vi "Simulation - Kopie.vi"() -> ()   [LabVIEW 2014]
uses:
  <vilib>/Simulation/Scripting/Companion Diagram/SimConfigNode/SimParams.ctl
  <vilib>/Simulation/Scripting/Companion Diagram/SimConfigNode/_simSolvers.ctl
  <vilib>/Simulation/Implementation/Shared/SIMSCR Execution Mode.ctl
  <vilib>/Platform/TimedLoop/XDataNode/timing_clust.ctl
  <vilib>/Platform/TimedLoop/XDataNode/nitl_modes.ctl
  <vilib>/Platform/TimedLoop/XDataNode/wakeup.ctl
  <vilib>/Simulation/Param Hierarchy/Typedefs/SIMPH Param Control Actions.ctl
  <vilib>/Analysis/3filter.llb/Filter Passband Type.ctl
  <vilib>/Simulation/Implementation/Shared/NILVSim_ParamChanged.vi
  <vilib>/Simulation/Implementation/Shared/NILVSim_FinishedLate.vi
  <vilib>/Simulation/Implementation/Shared/NILVSIM_BeginStep.vi
  <vilib>/Simulation/Utility/Implementation/SIM Halt.vi
  <vilib>/Simulation/SignalArithmetic/Implementation/NILVSim Gain.llb/SIM Gain (scalar).vi
  <vilib>/Simulation/ContinuousLinear/Implementation/NILVSim Transfer Function.llb/SIM Transfer Function Distributor (SISO).vi
  <vilib>/Simulation/Implementation/Shared/SIM Is Init or Final Stage.vi
  <vilib>/Simulation/ContinuousLinear/Implementation/NILVSim State Space.llb/SIM State Space Distributor (CD).vi
  <vilib>/Simulation/Nonlinear/Implementation/NILVSim Quantizer.llb/SIM Quantizer (scalar).vi
  <vilib>/Simulation/ContinuousLinear/Implementation/NILVSim Transfer Function.llb/SIM Transfer Function Collector (SISO).vi
  <vilib>/Simulation/SignalArithmetic/Implementation/NILVSim Gain.llb/SIM Gain (vector,MatrixGain).vi
  <vilib>/Simulation/Nonlinear/Implementation/NILVSim Saturation.llb/SIM Saturation (scalar).vi
  <vilib>/Simulation/ContinuousLinear/Implementation/NILVSim State Space.llb/SIM State Space Collector (CD).vi
  <vilib>/Simulation/SignalArithmetic/Implementation/NILVSim Gain.llb/SIM Gain (vector).vi
  <vilib>/Simulation/Implementation/Shared/NILVSim_Manager.vi
  <vilib>/Utility/error.llb/Clear Errors.vi
  <vilib>/Simulation/Implementation/Shared/NILVSim_FinalizeModel.vi
  <vilib>/addons/Control Design/_Model Construction/Model Creation.llb/Model Creation SubVI/cd_Create State Space Model.vi
  <vilib>/addons/Control Design/_Utility/Model Viewer.llb/Model Viewer SubVI/cd_Draw State-Space Equation (SS).vi
  <vilib>/Simulation/Implementation/Shared/SIM Unbundle Sim Info.vi
  <vilib>/Simulation/Implementation/Shared/SIMSH Read Queue.vi
  <vilib>/Simulation/Implementation/Shared/NILVSim_Initialize.vi
  <vilib>/addons/Control Design/_State Feedback Control/State Feedback Control.llb/CD Linear Quadratic Regulator.vi
  <vilib>/addons/Control Design/_State Feedback Control/State Feedback Control.llb/State Feedback Control SubVis/cd_Linear Quadratic Regulator.vi
  <vilib>/ptbypt/Probability & Statistics.llb/Median PtByPt.vi
  <vilib>/Simulation/Utility/Implementation/NILVSim Get Time and IsAcceptedStep.vi
  <vilib>/ptbypt/Filters.llb/Butterworth Filter PtByPt.vi
  <vilib>/Simulation/Implementation/Shared/NILVSim_GetModelError.vi
  <vilib>/Simulation/Implementation/Shared/SIM Bundle Sim Info.vi
  <vilib>/Simulation/Scripting/Companion Diagram/SimConfigNode/SimDog.xnode
  Nichtlineares Pendelmodell Sub.vi
  LabView/Beobachter/Nichtlinearer Beobachter.vi
  <vilib>/Platform/TimedLoop/XDataNode/XDataNode.xnode
  <vilib>/addons/Control Design/_Model Construction/Model Typedefs.llb/CD State Space Model (MIMO).ctl
  <vilib>/addons/Control Design/_Model Construction/Model Typedefs.llb/CD General Elements.ctl
  <vilib>/Simulation/Implementation/XNodeFramework/SimXNode/SimX.xnode
  <vilib>/addons/Control Design/_Model Construction/NI_LinSys_Model Typedefs.lvlib
  <vilib>/addons/Control Design/_State Feedback Control/NI_CD_State Feedback Control.lvlib
  <vilib>/addons/Control Design/_Utility/NI_CD_Model Viewer.lvlib
  <vilib>/addons/Control Design/_Model Construction/NI_LinSys_Model Creation.lvlib
  <vilib>/Simulation/ContinuousLinear/Implementation/NILVSim State Space.llb/SIM State Space (CD).vi
  <vilib>/ptbypt/NI_PtbyPt.lvlib
  <vilib>/Analysis/NI_AALBase.lvlib
  <vilib>/Simulation/ContinuousLinear/Implementation/NILVSim Transfer Function.llb/SIM Transfer Function (SISO).vi
  <vilib>/Platform/TimedLoop/XDataNode/XDNodeRunTimeDep.lvlib
  <vilib>/Simulation/Implementation/Shared/NI_SIM_Implementation.lvlib
panel:
  in  "Kraftverstärkung":dbl=1.0
  in  "Winkelg._t0":dbl
  in  "Enum":enum16{"median", "kein", "pt2"}(ring)
  in  "Enc. resolution":dbl
  in  "low cutoff freq: fl":dbl=0.125 caption="Untere Grenzfreq: fl" format="%0.3f"
  in  "WG Regler":T1(ring)
  out "Winkelgeschw. geschätzt vs gesch.+gefiltert (abs. Fehler)":dbl(graph)
  in  "WG Aufschw.":T1(ring)
  out "geschätzt+gefiltert":dbl
  out "Cruise mode":i32(graph)=1
  out "Regler":i16(graph)=1
  in  "< Winkelgeschwindigkeit (rad)":dbl=1.0
  in  ">Winkel (Grad) AUS":dbl=15.0
  in  "<Winkel (Grad) EIN":dbl=10.0
  in  "k_eu (EIN)":dbl=0.02
  in  "k_el (AUS)":dbl=-0.1
  in  "k_eo (Energieoffset)":dbl=0.02
  in  "k_ce (Energiezufuhr)":dbl=5.0
  out "E kin":sgl(graph)=9.683897e-12
  out "E pot":sgl(graph)=-2.0909203e-09
  out "E gesamt":sgl(graph)=-2.0812365e-09
  in  "Position_t0 (m)":dbl
  out "Kraft in N":dbl=0.019527387596300915
  out "winkelgesch Geschätzt":dbl=-3.1760654462499827e-05
  out "Winkelgesch. Simuliert":dbl=-3.1760671506439986e-05
  out "Winkel  (rad)":dbl=6.283279545734089
  out "Geschwindigkeit":dbl=-0.0005385174095775639
  out "Position":dbl=-499.86322344217655
  out "Regler EIN":bool=TRUE
  in  "k_v (velocity well)":dbl=1.0
  in  "k_x (cart well)":dbl=2.5
  in  "k_e (Energiezufuhr)":dbl=2.2
  in  "Aufschwingen":bool=TRUE
  in  "Strecke":T2(ring)
  out "State-Space Equation":picture
  out "Position (mm)":cluster{"output":dbl, "output":dbl}(graph)={"output"=-500.0, "output"=-499.86322344217655}
  out "Winkel (Grad)":T3(graph)
  out "Kraft (N)":dbl(graph)=0.019527387596300915
  out "Geschwindigkeit":dbl(graph)=-0.0005385174095775639
  out "Winkelgeschwindigkeit":T4(graph)
  out "K":dbl[][](array[numeric])=[[-100.00000000000013, -103.52787904437508, -700.9266185415707, -140.20536929914581]] format="%.2f"
  in  "Q":dbl[][](array[numeric])=[[100.0, 0.0, 0.0, 0.0], [0.0, 1.0, 0.0, 0.0], [0.0, 0.0, 100.0, 0.0], [0.0, 0.0, 0.0, 1.0]] format="%.2f"
  in  "R":dbl[][](array[numeric])=[[0.01]] format="%.2f"
  in  "Regler":bool=TRUE
  in  "Winkel_t0 (Grad)":dbl=180.0
  in  "Sollwert Amplitude (mm)":dbl=-500.0
  in  "Stop Button":bool
  # "Anfangswerte"
  # "Aufschwingparameter"
  # "Umschalten auf Cruise Mode. Energiegrenzen in J."
  # "Umschalten auf Regler"
  # "LQR Regler"
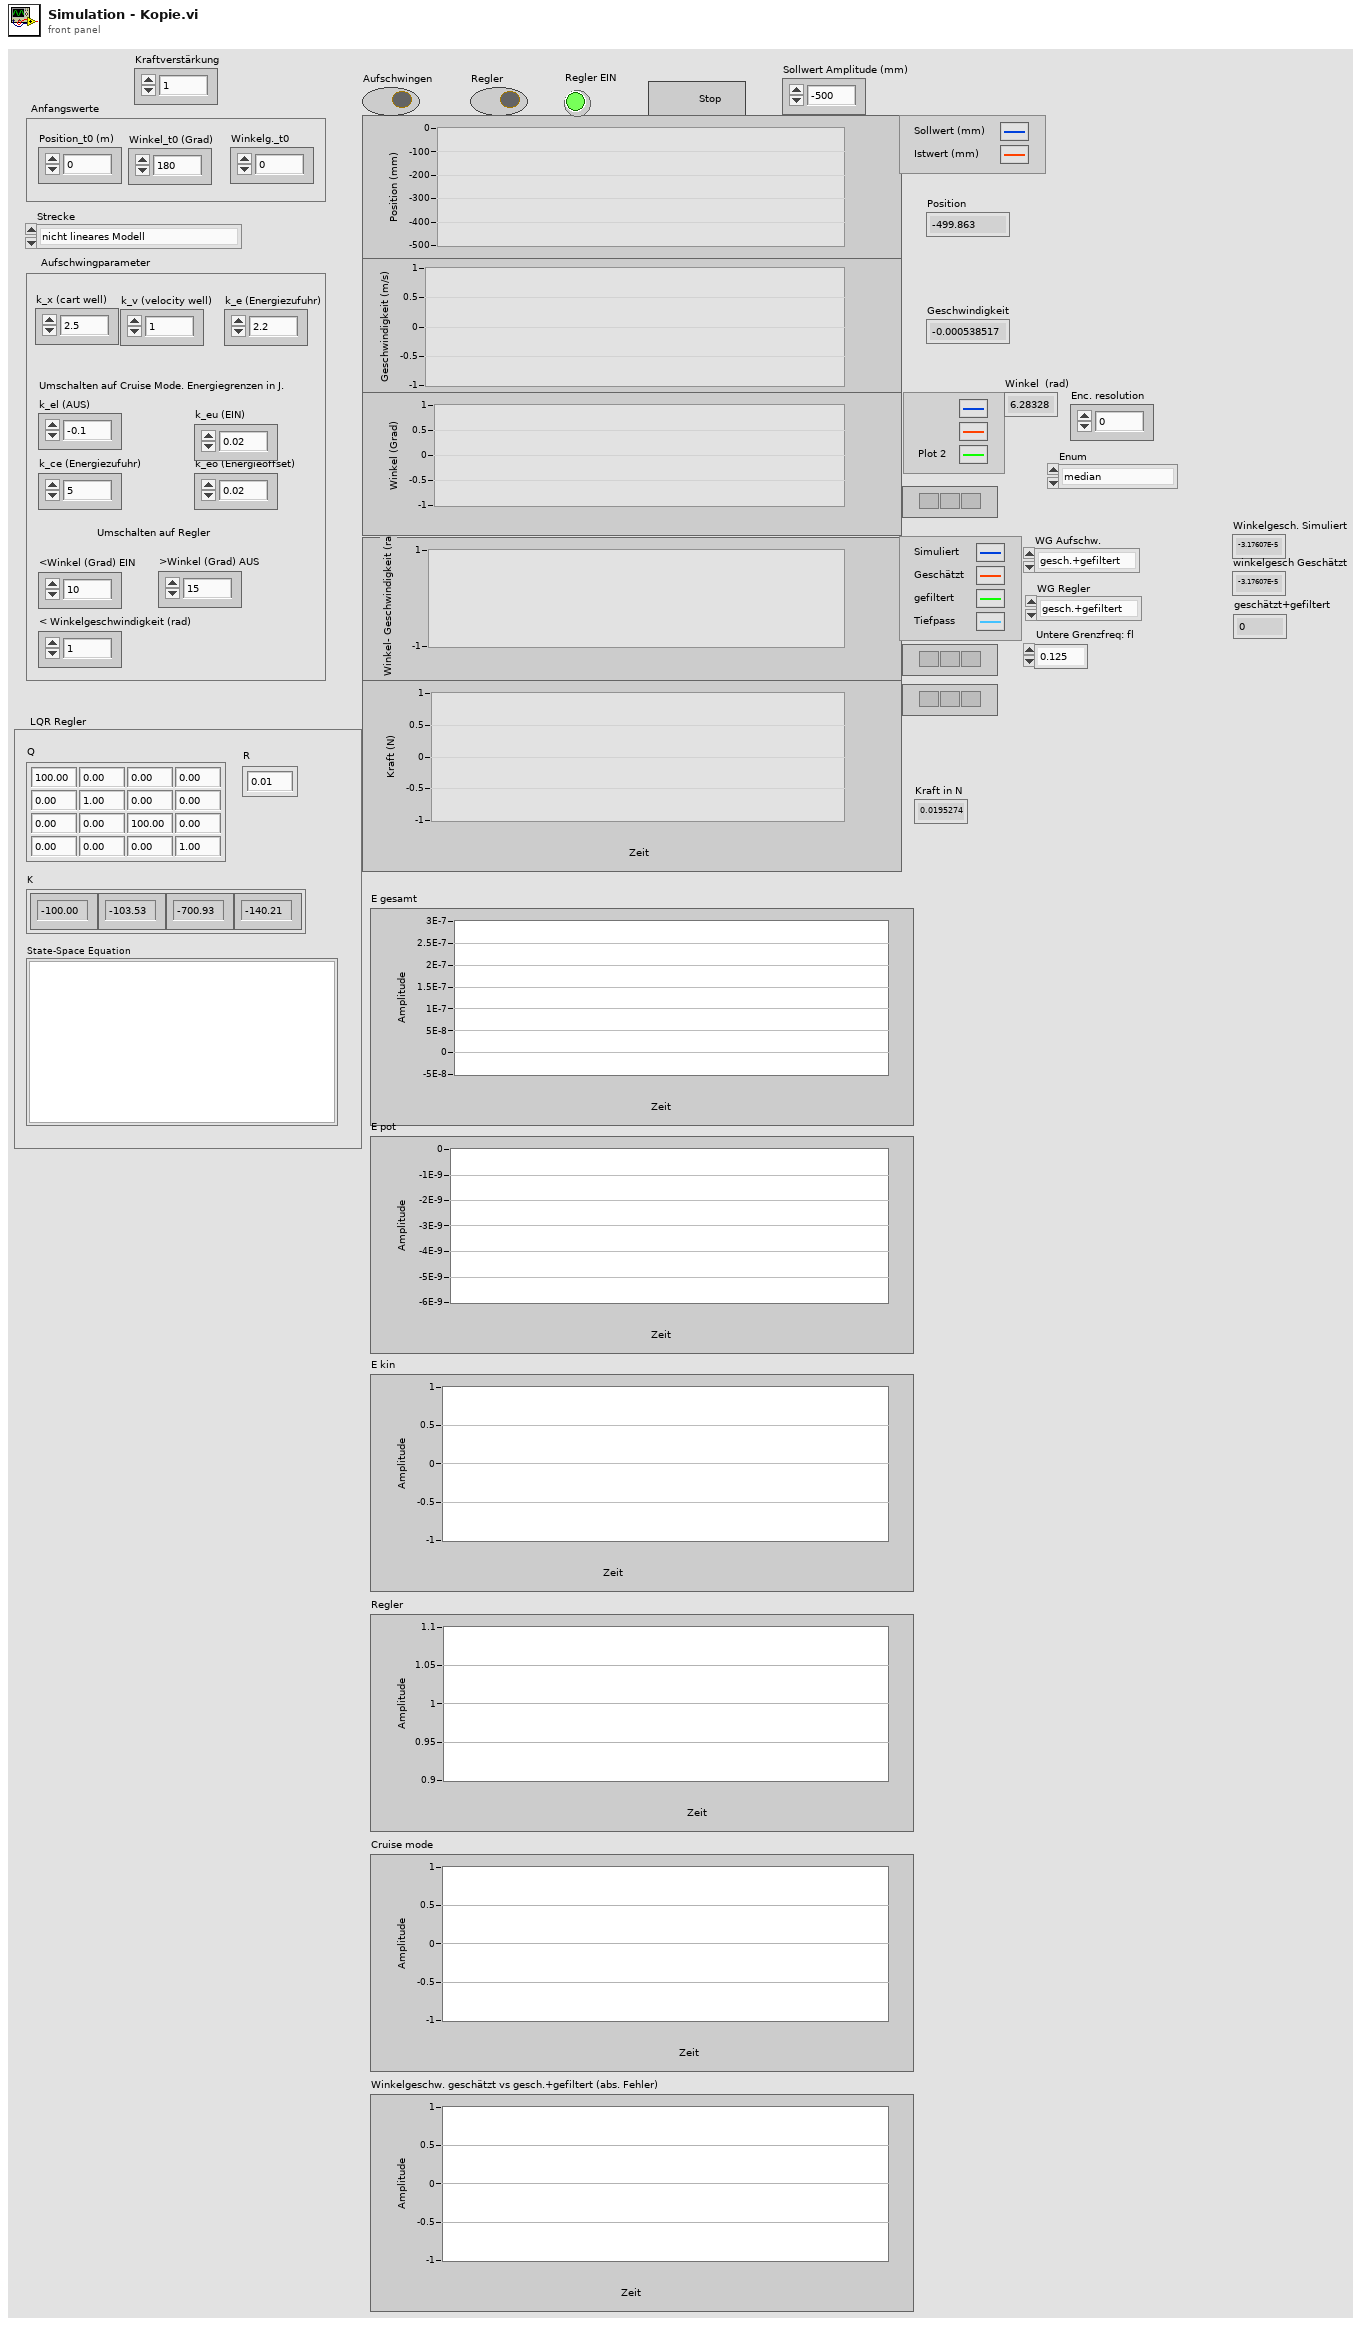
[diagram p1: front panel]
types:
  T1 = enum16{"gesch.+gefiltert", "geschätzt", "simuliert"}
  T2 = enum16{"nicht lineares Modell", "lineares Modell"}
  T3 = cluster{"output":dbl, "output y(t)":dbl, "median":dbl}
  T4 = cluster{"Winkelgesch":dbl, "x4_":dbl, "median":dbl, "Filtered x":dbl}
  T5 = typedef "NI_LinSys_Model Typedefs.lvlib/CD State Space Model (MIMO).ctl" = cluster{"properties":T6, "A":dbl[][], "B":dbl[][], "C":dbl[][], "D":dbl[][], "StateNames":string[], "Transport Delay":dbl[][]}
  T6 = typedef "NI_LinSys_Model Typedefs.lvlib/CD General Elements.ctl" = cluster{"Model name":string, "Input names":string[], "Output names":string[], "Input Delays":dbl[], "Output Delays":dbl[], "Sampling Time":dbl, "Notes":string}
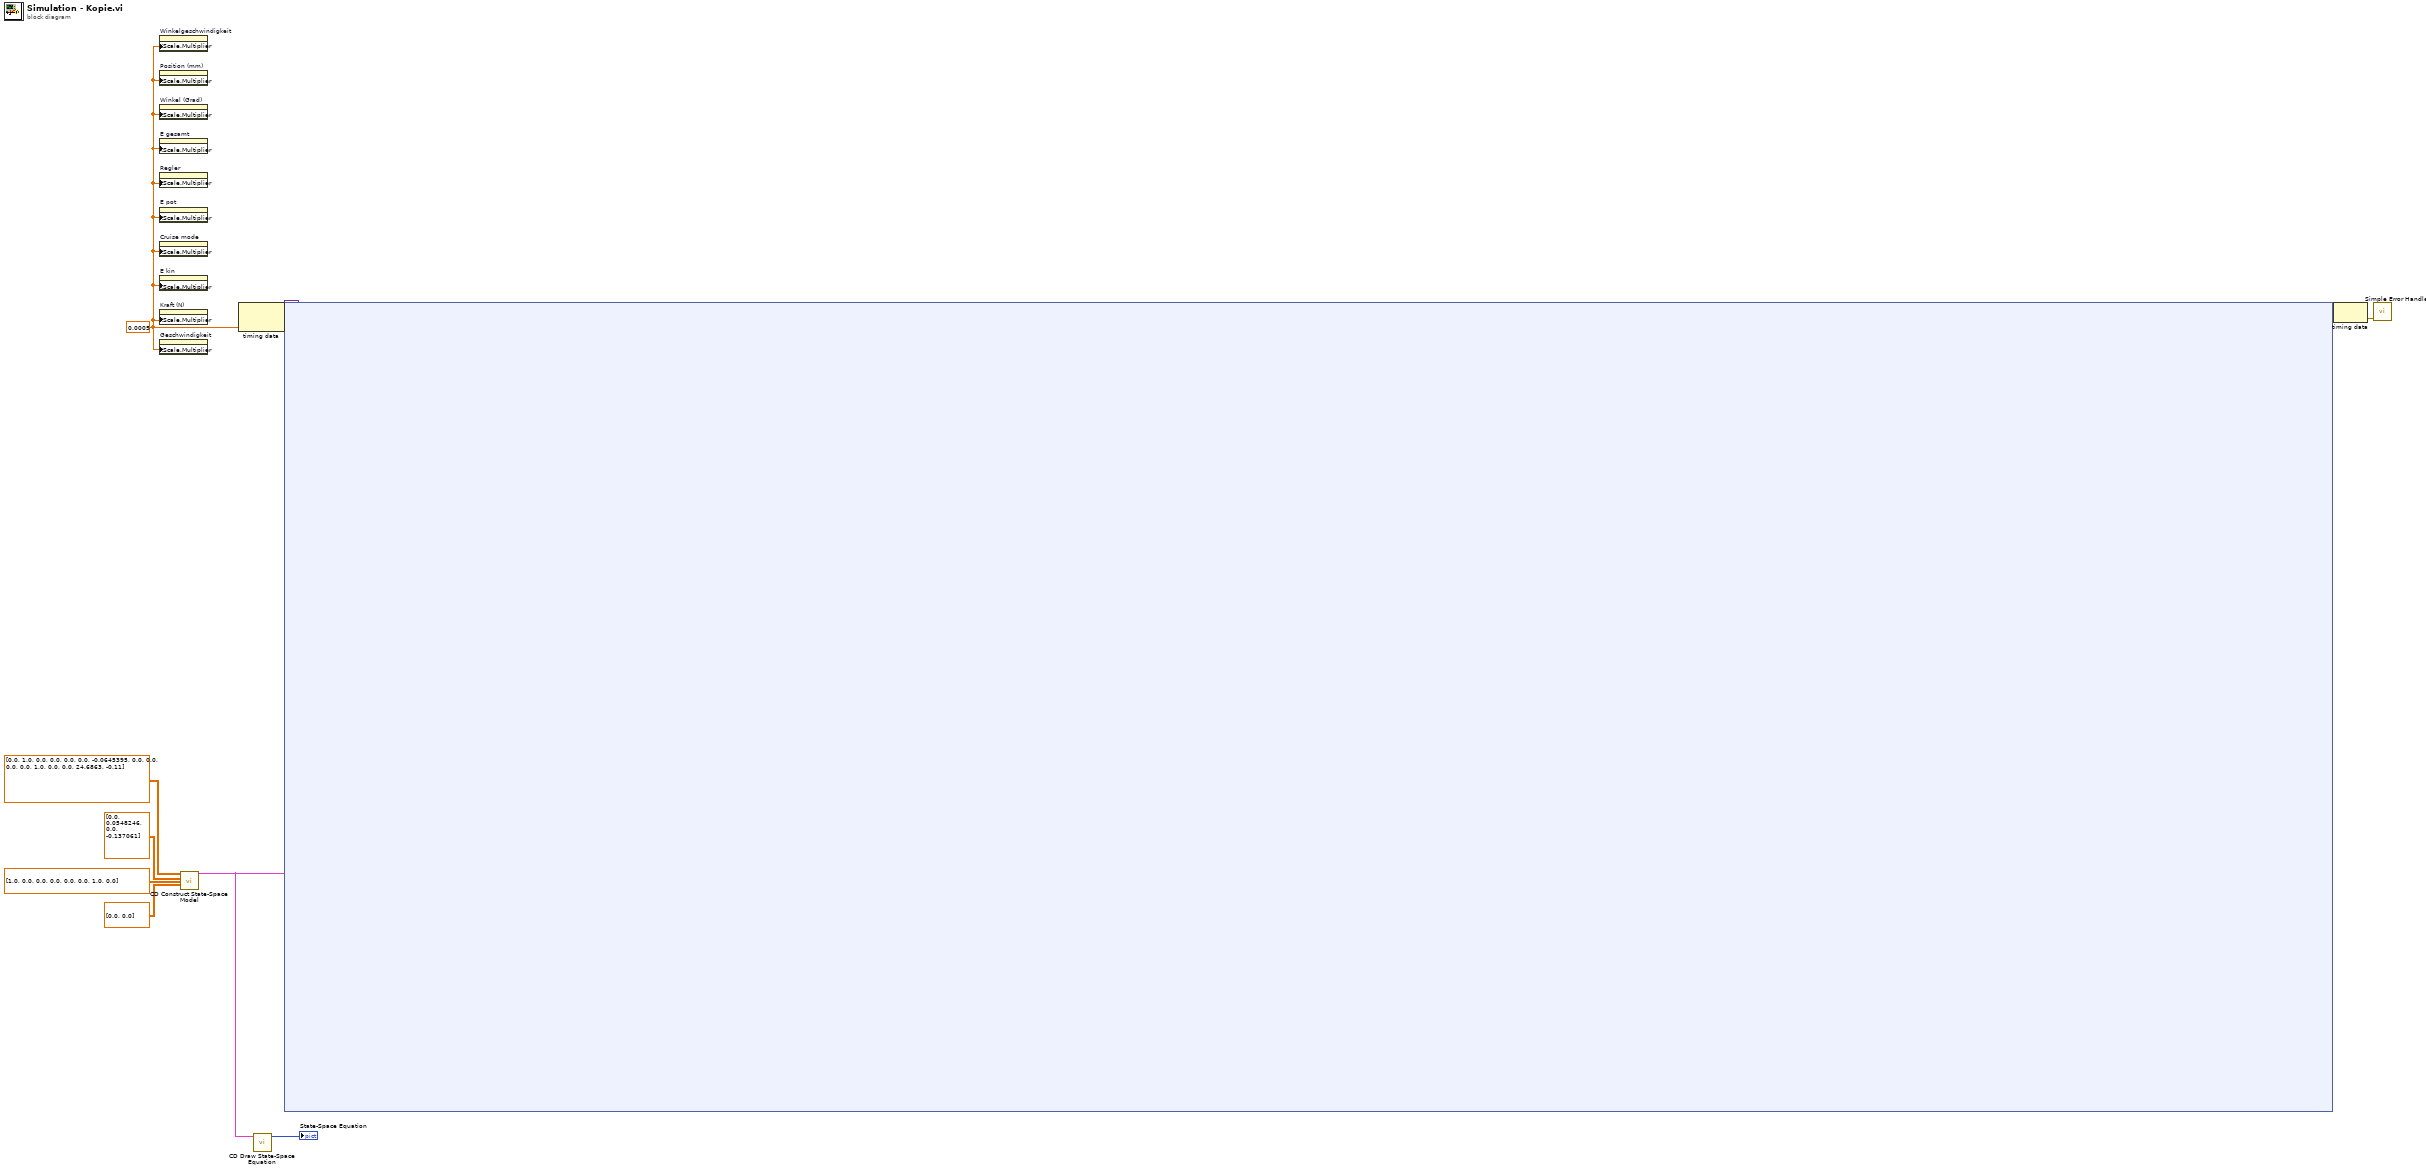
[diagram p0: block diagram]
diagram:
  w1 = 0.0005 ("Step Size (s)")
  n1 = property on="Winkelgeschwindigkeit" class="SVDiagr (strikt)"("XScale.Multiplier"=w1) -> ()  [unwired: 2 in, 2 out]
  n2 = property on="Position (mm)" class="SVDiagr (strikt)"("XScale.Multiplier"=w1) -> ()  [unwired: 2 in, 2 out]
  n3 = property on="Winkel (Grad)" class="SVDiagr (strikt)"("XScale.Multiplier"=w1) -> ()  [unwired: 2 in, 2 out]
  n4 = property on="E gesamt" class="SVDiagr (strikt)"("XScale.Multiplier"=w1) -> ()  [unwired: 2 in, 2 out]
  n5 = property on="Regler" class="SVDiagr (strikt)"("XScale.Multiplier"=w1) -> ()  [unwired: 2 in, 2 out]
  n6 = property on="E pot" class="SVDiagr (strikt)"("XScale.Multiplier"=w1) -> ()  [unwired: 2 in, 2 out]
  n7 = property on="Cruise mode" class="SVDiagr (strikt)"("XScale.Multiplier"=w1) -> ()  [unwired: 2 in, 2 out]
  n8 = property on="E kin" class="SVDiagr (strikt)"("XScale.Multiplier"=w1) -> ()  [unwired: 2 in, 2 out]
  n9 = property on="Kraft (N)" class="SVDiagr (strikt)"("XScale.Multiplier"=w1) -> ()  [unwired: 2 in, 2 out]
  n10 = property on="Geschwindigkeit" class="SVDiagr (strikt)"("XScale.Multiplier"=w1) -> ()  [unwired: 2 in, 2 out]
  n11 = call-poly <vilib>:"CD Construct State-Space Model.vi"("A"=dbl[][] [[0.0, 1.0, 0.0, 0.0], [0.0, 0.0, -0.0645395, 0.0], [0.0, 0.0, 0.0, 1.0], [0.0, 0.0, 24.6863, -0.11]], "B"=dbl[][] [[0.0], [0.0548246], [0.0], [-0.137061]], "C"=dbl[][] [[1.0, 0.0, 0.0, 0.0], [0.0, 0.0, 1.0, 0.0]], "D"=dbl[][] [[0.0], [0.0]]) -> ("State-Space Model"=w2:T5)  [unwired: 10 in, 1 out]
  n12 = node-c288(w1) -> (w10:variant)  [unwired: 1 in]
  n13 = call-poly <vilib>:"CD Draw State-Space Equation.vi"("State-Space Model"=w2) -> ("Equation"=→"State-Space Equation":picture)  [unwired: 8 in, 2 out]
  n14 = node-c254 ("Control & Simulation Loop")(w10, w2) -> (w9:variant)
  n15 = node-c288(w9) -> (w8:errorcluster)
  n16 = call <vilib>:"Simple Error Handler.vi"("error in (no error)"=w8) -> ()  [unwired: 4 in, 5 out]
